vi "Min.vi"(8 "error in (no error)":errorcluster, 10 "Numeric":dbl, 11 "Contador Binario in":refnum<class "Contador Binario.lvclass">) -> (0 "error out":errorcluster, 3 "Contador Binario out":refnum<class "Contador Binario.lvclass">)   [LabVIEW 2020, in "Contador Binario.lvlib" / "Contador Binario.lvclass"]
uses:
  Contador Binario.lvclass
  Contador Binario.lvclass/Contador Binario.ctl
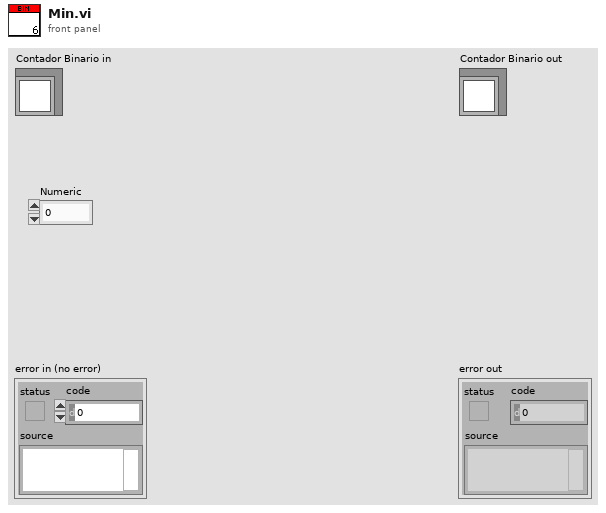
[diagram p1: front panel]
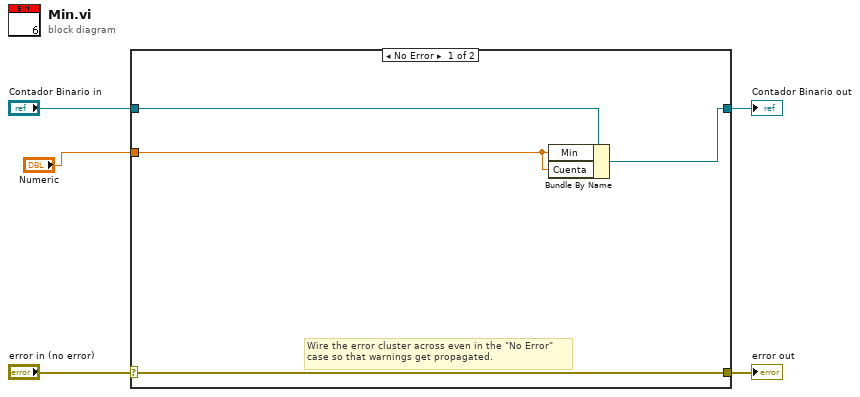
[diagram p0: block diagram]
diagram:
  n1 = case shown="No Error" "error in (no error)" {
    selector: "error in (no error)" -> [w9 w11]
    tunnel: [w9 w11] -> w4
    tunnel: [w7 w10] -> w2
    tunnel: "Contador Binario in" -> [w8 w10]
    tunnel: "Numeric" -> [w6 _]
    frame No Error {
      # "Wire the error cluster across even in the \"No Error\"\ncase so that warnings get propagated."
      n2 = Bundle By Name(cluster=w8, "Min"=w6, "Cuenta"=w6) -> (w7:refnum<class "Contador Binario.lvclass">)
    }
    frame Error {
    }
  }
  "error out" <- w4
  "Contador Binario out" <- w2
